vi "FPGA Close Outlet.vi"(0 "PV":fxp<+/-,21,-4>, 5 "SP Close Outlet":fxp<+/-,21,-4>, 7 "Enable Close Outlet":bool, 9 "Cycles to Filter":u16=5, 12 "#DO 1":T1=6 items=["DO 0 [KP1] [M12]", "DO 1 [ON KP2] [M21]", "DO 2 [ON KP3] [M24]", "DO 3 [WATER Y18.1 [DO3]]", "DO 4 [WATER Y18.2 [DO4]]", "DO 5 [KP6 Y29.1 33.7]", "DO 6 [KP7 Y29.2 33.8]", "DO 7 [KP8 Y29.3 33.9]", "DO 8 [KP9 Y29.4  33.12]", "DO 9 [KP10 Y29.5 33.1]", "DO 10 [KP11 Y29.6 33.2]", "DO 11 [KP12 Y29.7  33.13]", "DO 12 [KP13 Y29.8  33.11]", "DO 13 [KP14 Y29.9 33.10]", "DO 14 [KP15 Y29.10  33.6]", "DO 15 [KP16 Y29.11  33.5]", "DO 16 [KP17 Y29.12  33.4]", "DO 17 [KP18 Y29.13 33.3]", "DO 18 [AIR KP19]", "DO 19 [STEP DRIVE EN KP20]", "DO 20 [KP21 Y44.1 OPEN]", "DO 21 [ KP22 Y44.1 CLOSE]", "DO 22 [ KP23 Y44.2 OPEN]", "DO 23", "DO 24 [STEP DRIVE 1]", "DO 25 [STEP DRIVE 2]"], 13 "#DO 2":T1=17 items=["DO 0 [KP1] [M12]", "DO 1 [ON KP2] [M21]", "DO 2 [ON KP3] [M24]", "DO 3 [WATER Y18.1 [DO3]]", "DO 4 [WATER Y18.2 [DO4]]", "DO 5 [KP6 Y29.1 33.7]", "DO 6 [KP7 Y29.2 33.8]", "DO 7 [KP8 Y29.3 33.9]", "DO 8 [KP9 Y29.4  33.12]", "DO 9 [KP10 Y29.5 33.1]", "DO 10 [KP11 Y29.6 33.2]", "DO 11 [KP12 Y29.7  33.13]", "DO 12 [KP13 Y29.8  33.11]", "DO 13 [KP14 Y29.9 33.10]", "DO 14 [KP15 Y29.10  33.6]", "DO 15 [KP16 Y29.11  33.5]", "DO 16 [KP17 Y29.12  33.4]", "DO 17 [KP18 Y29.13 33.3]", "DO 18 [AIR KP19]", "DO 19 [STEP DRIVE EN KP20]", "DO 20 [KP21 Y44.1 OPEN]", "DO 21 [ KP22 Y44.1 CLOSE]", "DO 22 [ KP23 Y44.2 OPEN]", "DO 23", "DO 24 [STEP DRIVE 1]", "DO 25 [STEP DRIVE 2]"]) -> ()   [LabVIEW 2019]
uses:
  TypeDef/DO index.ctl
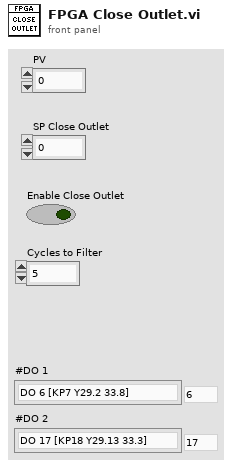
[diagram p1: front panel]
types:
  T1 = typedef "DO index.ctl" = u8
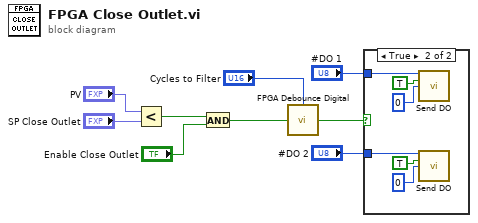
[diagram p0: block diagram]
diagram:
  n1 = Less?(x="PV", y="SP Close Outlet") -> (x < y?=w3:bool)
  n2 = And(x=w3, y="Enable Close Outlet") -> (x .and. y?=w2:bool)
  n3 = call "FPGA Debounce Digital.vi"("Input Signal"=w2, "Cycles to Filter"="Cycles to Filter") -> ("Output Filtered Signal"=w1:bool)
  n4 = case shown="True" w1 {
    tunnel: "#DO 2" -> [_ w11]
    tunnel: "#DO 1" -> [_ w10]
    frame False {
    }
    frame True {
      n5 = call "Send DO.vi"("#DO"=w10, "value"=TRUE, "Time uSec"=u32 0) -> ()  [unwired: 13 in]
      n6 = call "Send DO.vi"("#DO"=w11, "value"=TRUE, "Time uSec"=u32 0) -> ()  [unwired: 13 in]
    }
  }
